vi "Initialize.vi"(7 "Serial Configuration":cluster{"Baud Rate":u32}={"Baud Rate"=9600} {"Baud Rate" items=["4800"=4800, "9600"=9600, "19200"=19200, "38400"=38400, "57600"=57600, "115200"=115200]}, 8 "error in (no error)":errorcluster, 9 "Reset (True)":bool=TRUE, 10 "ID Query (True)":bool=TRUE, 11 "VISA resource name":refnum<visa-resource-name>) -> (0 "error out":errorcluster, 3 "VISA resource name out":refnum<visa-resource-name>)   [LabVIEW 2020, in "BK Precision 911X Series.lvlib"]
doc: "Establishes communication with the instrument and optionally performs an instrument identification query and/or an instrument reset. It also places the instrument in a default state needed for other instrument driver operations. Therefore, call this VI before calling other instrument driver VIs for this instrument. Generally, you need to call the Initialize VI only once at the beginning of an application."
uses:
  BK Precision 911X Series.lvlib
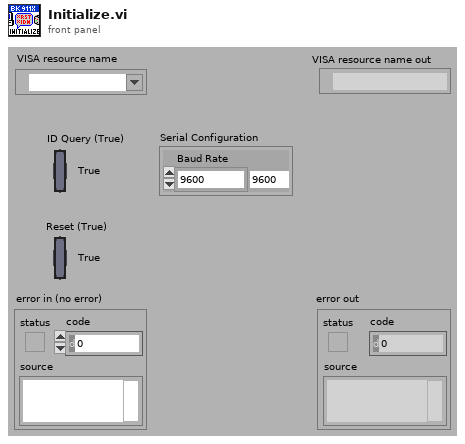
[diagram p1: front panel]
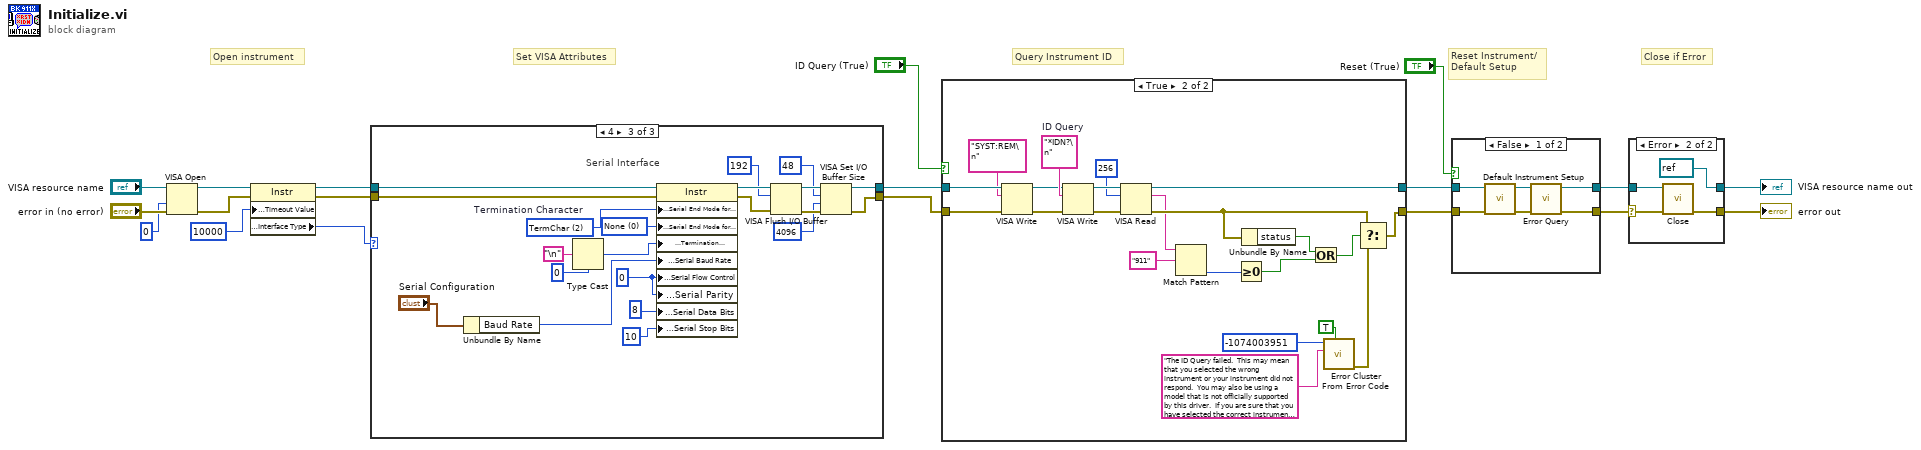
[diagram p0: block diagram]
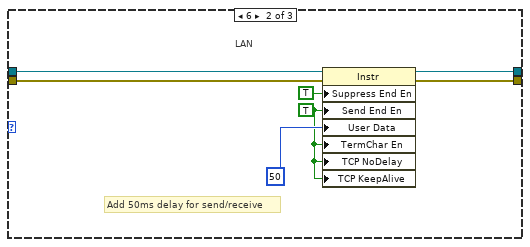
[diagram p3: hidden frame]
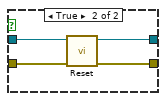
[diagram p5: hidden frame]
diagram:
  # "Set VISA Attributes"
  # "Close if Error"
  # "Query Instrument ID"
  # "Reset Instrument/\nDefault Setup"
  # "Open instrument"
  n1 = VISA Open(access mode=u32 0, error in (no error)="error in (no error)", VISA resource name="VISA resource name") -> (VISA resource name=w3:refnum<visa-resource-name>, error out=w2:errorcluster)  [unwired: 2 in]
  n2 = property class="Instr"(reference=w3, error in=w2, "General Settings:Timeout Value"=u32 10000) -> (reference out=w10:refnum<visa-resource-name>, error out=w9:errorcluster, "Interface Information:Interface Type"=w1:u16)
  n3 = case shown="4" w1 {
    tunnel: [w21 w24 w46] -> w12
    tunnel: [w20 w25 w43] -> w11
    tunnel: w10 -> [w21 w27 w48]
    tunnel: w9 -> [w20 w26 w49]
    frame 1, 7, Default {
      # "USBTMC and GPIB"
    }
    frame 6 {
      w22 = TRUE ("Message Based Settings:Send End Enable")
      # "Add 50ms delay for send/receive"
      # "LAN"
      n4 = property class="Instr"(reference=w27, error in=w26, "Suppress End En"=TRUE ("Message Based Settings:Suppress End Enable"), "Send End En"=w22, "User Data"=u32 50, "TermChar En"=w22, "TCP NoDelay"=w22, "TCP KeepAlive"=w22) -> (reference out=w24:refnum<visa-resource-name>, error out=w25:errorcluster)
    }
    frame 4 {
      w29 = u16 0 items=["None", "Last Bit", "TermChar", "Break"] ("Serial Settings:End Mode for Writes")
      w34 = 0
      w36 = u16 2 items=["None", "LastBit", "TermChar"]  # Termination Character
      # "Serial Interface"
      n5 = Unbundle By Name("Serial Configuration") -> ("Baud Rate"=w30:u32)
      n6 = Type Cast(type=u8 0, x="\n" ("Line Feed Constant")) -> (*(type *) &x=w35:u8)
      n7 = property class="Instr"(reference=w48, error in=w49, "Serial Settings:Serial End Mode for Reads"=w36, "Serial Settings:Serial End Mode for Writes"=w29, "Message Based Settings:Termination Character"=w35, "Serial Settings:Serial Baud Rate"=w30, "Serial Settings:Serial Flow Control"=w34, "Serial Settings:Serial Parity"=w34, "Serial Settings:Serial Data Bits"=8, "Serial Settings:Serial Stop Bits"=10) -> (reference out=w42:refnum<visa-resource-name>, error out=w45:errorcluster)
      n8 = VISA Flush I/O Buffer(VISA resource name=w42, mask (16)=u16 192, error in (no error)=w45) -> (VISA resource name out=w47:refnum<visa-resource-name>, error out=w44:errorcluster)
      n9 = VISA Set I/O Buffer Size(VISA resource name=w47, mask (16)=u16 48, size (4096)=u32 4096 ("size (0)"), error in (no error)=w44) -> (VISA resource name out=w46:refnum<visa-resource-name>, error out=w43:errorcluster)
    }
  }
  n10 = case shown="True" "ID Query (True)" {
    tunnel: [w50 w73] -> w18
    tunnel: [w51 w72] -> w19
    tunnel: w12 -> [w51 w55]
    tunnel: w11 -> [w50 w54]
    frame False {
    }
    frame True {
      w67 = "*IDN?\n"  # ID Query
      n11 = VISA Write(VISA resource name=w55, write buffer="SYST:REM\n", error in (no error)=w54) -> (VISA resource name out=w56:refnum<visa-resource-name>, error out=w57:errorcluster)  [unwired: 1 out]
      n12 = VISA Write(VISA resource name=w56, write buffer=w67, error in (no error)=w57) -> (VISA resource name out=w71:refnum<visa-resource-name>, error out=w70:errorcluster)  [unwired: 1 out]
      n13 = VISA Read(VISA resource name=w71, byte count=u32 256, error in (no error)=w70) -> (VISA resource name out=w72:refnum<visa-resource-name>, read buffer=w52:string, error out=w61:errorcluster)  [unwired: 1 out]
      n14 = Match Pattern(string=w52, regular expression="911") -> (offset past match=w62:i32)  [unwired: 1 in, 3 out]
      n15 = Greater Or Equal To 0?(x=w62) -> (x >= 0?=w59:bool)
      n16 = Unbundle By Name(w61) -> ("status"=w60:bool)
      n17 = Or(x=w60, y=w59) -> (x .or. y?=w58:bool)
      n18 = call <vilib>:"Error Cluster From Error Code.vi"("show call chain? (False)"=TRUE, "error message (\"\")"="The ID Query failed.  This may mean that you selected the wrong instrument or your instrument did not respond.  You may also be using a model that is not officially supported by this driver.  If you are sure that you have selected the correct instrument and it is responding, try disabling the ID Query." ("Source (VI Name)"), "error code (0)"=-1074003951 ("Code")) -> ("error out"=w66:errorcluster)  [unwired: 6 in]
      n19 = Select(t=w61, s=w58, f=w66) -> (s? t:f=w73:errorcluster)
    }
  }
  n20 = case shown="False" "Reset (True)" {
    tunnel: w18 -> [w78 w80]
    tunnel: [w75 w83] -> w4
    tunnel: w19 -> [w79 w81]
    tunnel: [w76 w82] -> w5
    frame False {
      n21 = call "Default Instrument Setup.vi"("error in (no error)"=w78, "VISA resource name"=w79) -> ("error out"=w74:errorcluster, "VISA resource name out"=w77:refnum<visa-resource-name>)  [unwired: 8 in]
      n22 = call "Error Query.vi"("error in (no error)"=w74, "VISA resource name"=w77) -> ("error out"=w75:errorcluster, "VISA resource name out"=w76:refnum<visa-resource-name>)  [unwired: 6 in, 2 out]
    }
    frame True {
      n23 = call "Reset.vi"("error in (no error)"=w80, "VISA resource name"=w81) -> ("error out"=w83:errorcluster, "VISA resource name out"=w82:refnum<visa-resource-name>)  [unwired: 8 in]
    }
  }
  n24 = case shown="Error" w4 {
    selector: w4 -> [w84 w87]
    tunnel: w5 -> [w85 w88]
    tunnel: [w85 refnum<visa-resource-name> refnum ("VISA resource name out")] -> w7
    tunnel: [w84 w89] -> w6
    frame No Error {
    }
    frame Error {
      n25 = call "Close.vi"("error in (no error)"=w87, "VISA resource name"=w88) -> ("error out"=w89:errorcluster)  [unwired: 9 in]
    }
  }
  "VISA resource name out" <- w7
  "error out" <- w6
